vi "Bluetooth inicjalizacja.vi"(11 "time limit ms (10000)":i32) -> (0 "error out":errorcluster, 1 "service list":T1(array[cluster]), 2 "Number of devices":u16, 3 "Bluetooth Network Connection out":refnum<k31>, 4 "channel":u16, 5 "Device Name":string)   [LabVIEW 2012]
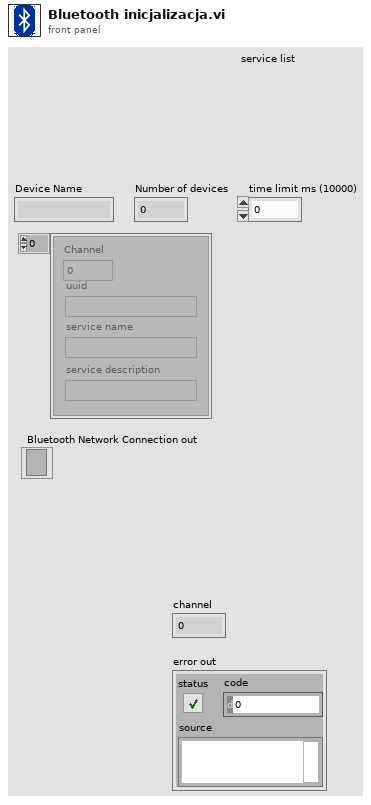
[diagram p1: front panel]
types:
  T1 = cluster{"Channel":u16, "uuid":string, "service name":string, "service description":string}[]
  T2 = cluster{"Address":string, "Device Name":string}[]
  T3 = cluster{"channel":u16, "uuid":string, "service name":string, "service description":string}[]
  T4 = cluster{"channel":u16, "uuid":string, "service name":string, "service description":string}
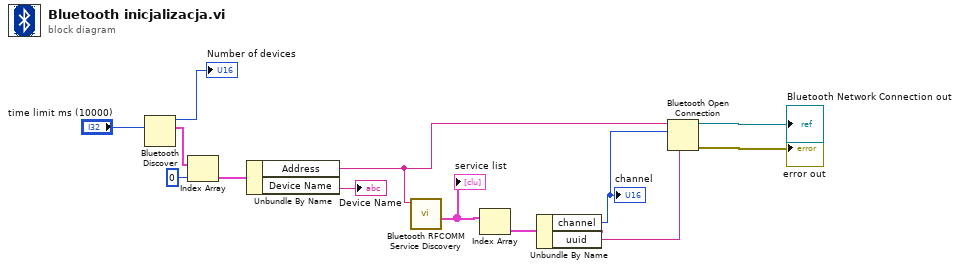
[diagram p0: block diagram]
diagram:
  n1 = Bluetooth Discover(10:"time limit ms (10000)") -> (2:w3:T2, 3:→"Number of devices":u16)  [unwired: 1 in, 1 out]
  n2 = Index Array(array=w3, index=0) -> (element=w5:cluster{"Address":string, "Device Name":string})
  n3 = Unbundle By Name(w5) -> ("Address"=w11:string, "Device Name"=→"Device Name":string)
  n4 = call <vilib>:"Bluetooth RFCOMM Service Discovery.vi"("address in"=w11) -> ("service list"=w7:T3)  [unwired: 3 in, 3 out]
  "service list" <- w7
  n5 = Index Array(array=w7) -> (element=w8:T4)  [unwired: 1 in]
  n6 = Unbundle By Name(w8) -> ("channel"=w10:u16, "uuid"=w9:string)
  "channel" <- w10
  n7 = Bluetooth Open Connection(6:w9, 10:w10, 11:w11) -> (0:→"error out":errorcluster, 3:→"Bluetooth Network Connection out":refnum<k31>)  [unwired: 2 in]
